vi "Control System.vi"() -> ()   [LabVIEW 2020]
panel:
  in  "Stop":bool
  out "Waveform Chart":cluster{dbl, "Set Point":dbl}(graph)
  in  "Set Point":dbl=10.0
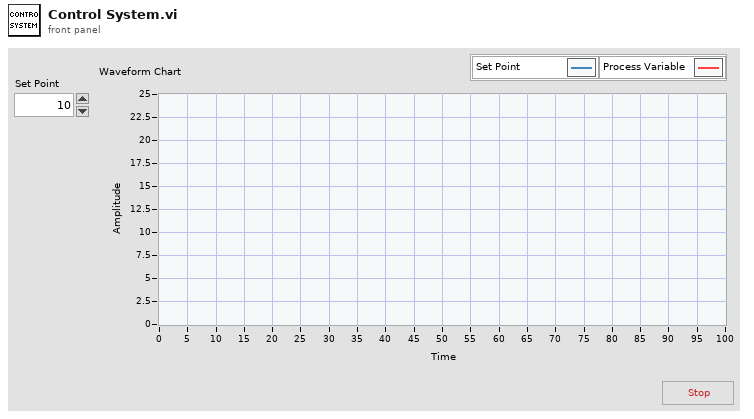
[diagram p1: front panel]
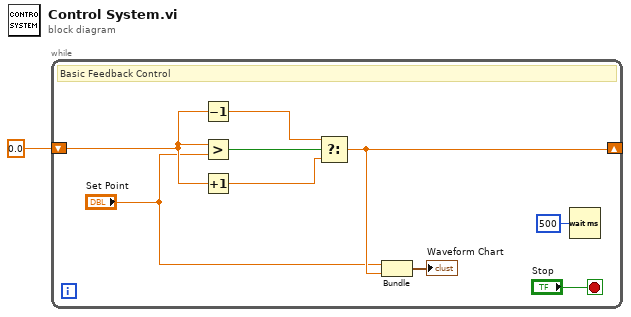
[diagram p0: block diagram]
diagram:
  n1 = while {
    shift-right: [w6] -> _
    shift-left: 0.0 ("Set Point") -> [w8]
    stop <- "Stop" stop-if-true
    # "Basic Feedback Control"
    n2 = Decrement(x=w8) -> (x-1=w9:dbl)
    n3 = Greater?(x=w8, y="Set Point") -> (0:w10:bool)
    n4 = Increment(x=w8) -> (x+1=w7:dbl)
    n5 = Select(t=w9, s=w10, f=w7) -> (s? t:f=w6:dbl)
    n6 = Bundle("Set Point"="Set Point", w6) -> (→"Waveform Chart":cluster{"Set Point":dbl, dbl})  [unwired: 1 in]
    n7 = Wait (ms)(milliseconds to wait=u32 500) -> ()  [unwired: 1 out]
  }
